vi "Splash Screen.vi"() -> ()   [LabVIEW 2026, in "CI Tests Launcher.lvlib"]
doc: "This is the top-level VI of this application. When it runs, it behaves like the splash screen many applications use to keep the user occupied while the application loads into memory. This application is quite small, so there is little overhead, which would make the splash screen just flash for a moment. Because that flash is distracting, there is a three-second delay inserted into this VI so that it stays up for a little bit. \n\nThis VI uses a delay-loaded subVI call to load the rest of the application. This trick ensures that the splash screen can load instantly regardless of how large the rest of the VI hierarchy gets, and the loading of the rest of the VIs becomes one step in the load process."
uses:
  CI Tests Launcher.lvlib
  CI Tests/CI Tests/Load App.vi
  CI Tests/CI Tests/CI Tests.lvclass
panel:
  out "Waiting Lights":T1
  out "Application Name":string
  out "Current Action":string caption="Current action:"
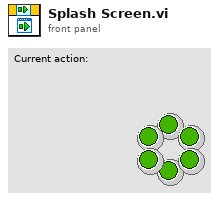
[diagram p1: front panel]
types:
  T1 = cluster{"wait 1":bool, "wait 2":bool, "wait 3":bool, "wait 4":bool, "wait 5":bool, "wait 6":bool}
  T2 = cluster{"[0]":bool, "[1]":bool, "[2]":bool, "[3]":bool, "[4]":bool, "[5]":bool}
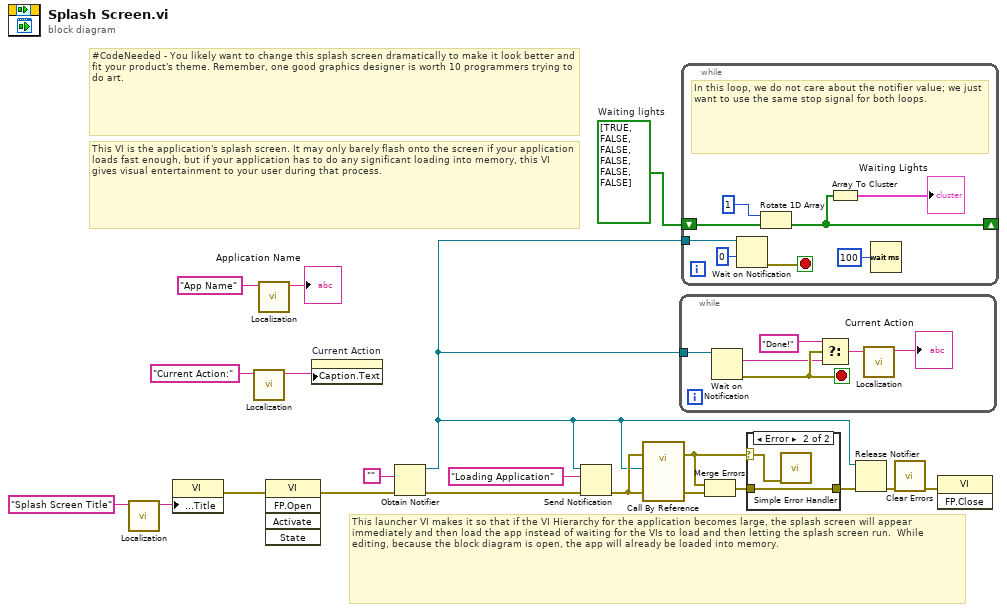
[diagram p0: block diagram]
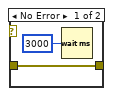
[diagram p2: hidden frame]
diagram:
  w10 = bool[] [TRUE, FALSE, FALSE, FALSE, FALSE, FALSE]  # Waiting lights
  # "#CodeNeeded - You likely want to change this splash screen dramatically to make it look better and fit your product's theme. Remember, one good graphics designer is worth 10 programmers trying to do art."
  # "This VI is the application's splash screen. It may only barely flash onto the screen if your application loads fast enough, but if your application has to do any significant loading into memory, this VI gives visual entertainment to your user during that process."
  # "This launcher VI makes it so that if the VI Hierarchy for the application becomes large, the splash screen will appear immediately and then load the app instead of waiting for the VIs to load and then letting the splash screen run.  While editing, because the block diagram is open, the app will already be loaded into memory."
  n1 = call "Localization.vi"("Unlocalized"="Splash Screen Title" ("Window Title")) -> ("Localized"=w20:string)  [unwired: 10 in]
  n2 = property class="VI"("Front Panel.Title"=w20) -> (error out=w2:errorcluster)  [unwired: 2 in, 1 out]
  n3 = call "Localization.vi"("Unlocalized"="Current Action:" ("Window Title")) -> ("Localized"=w6:string)  [unwired: 10 in]
  n4 = call "Localization.vi"("Unlocalized"="App Name") -> ("Localized"=→"Application Name":string)  [unwired: 10 in]
  n5 = invoke class="VI" method="FP.Open"(error in=w2) -> (error out=w1:errorcluster)  [unwired: 4 in, 4 out]
  n6 = property on="Current Action" class="Str"("Caption.Text"=w6) -> ()  [unwired: 2 in, 2 out]
  n7 = Obtain Notifier(notification data type="", error in (no error)=w1) -> (notifier out=w14:refnum<notifier>, error out=w8:errorcluster)  [unwired: 2 in, 1 out]
  n8 = Send Notification(notification="Loading Application", notifier=w14, error in (no error)=w8) -> (error out=w15:errorcluster)  [unwired: 1 out]
  n9 = call-by-ref "?"(error in=w15, 8:"error in (no error)"=w15, "Status Notifier"=w14) -> (error out=w3:errorcluster, 0:"error out"=w18:errorcluster)  [unwired: 10 in, 1 out]
  n10 = while {
    tunnel: w14 -> [w25]
    stop <- w24 stop-if-true
    n11 = Wait on Notification(notifier=w25) -> (notification=w22:string, error out=w24:errorcluster)  [unwired: 3 in, 2 out]
    n12 = Select(t="Done!" ("notification"), s=w24, f=w22) -> (s? t:f=w21:string)
    n13 = call "Localization.vi"("Unlocalized"=w21) -> ("Localized"=→"Current Action":string)  [unwired: 10 in]
  }
  n14 = while {
    shift-right: [w28] -> _
    shift-left: w10 -> [w30]
    tunnel: w14 -> [w32]
    stop <- w34 stop-if-true
    # "In this loop, we do not care about the notifier value; we just want to use the same stop signal for both loops."
    n15 = Wait on Notification(notifier=w32, timeout in ms (-1)=0) -> (error out=w34:errorcluster)  [unwired: 2 in, 3 out]
    n16 = Rotate 1D Array(1:w30, 2:1 ("n")) -> (0:w28:bool[])
    n17 = Array To Cluster(array=w28) -> (cluster=→"Waiting Lights":T2)
    n18 = Wait (ms)(milliseconds to wait=u32 100) -> ()  [unwired: 1 out]
  }
  n19 = Merge Errors(w3, w18) -> (w4:errorcluster)
  n20 = case shown="Error" w3 {
    tunnel: [w36 w37] -> w5
    tunnel: w4 -> [w36 w37]
    selector: w3 -> [_ w38]
    frame No Error {
      n21 = Wait (ms)(milliseconds to wait=u32 3000) -> ()  [unwired: 1 out]
    }
    frame Error {
      n22 = call <vilib>:"Simple Error Handler.vi"("error in (no error)"=w38) -> ()  [unwired: 4 in, 5 out]
    }
  }
  n23 = Release Notifier(notifier=w14, error in (no error)=w5) -> (error out=w17:errorcluster)  [unwired: 1 in, 2 out]
  n24 = call <vilib>:"Clear Errors.vi"("error in (no error)"=w17) -> ("error out"=w9:errorcluster)  [unwired: 5 in, 1 out]
  n25 = invoke class="VI" method="FP.Close"(error in=w9) -> ()  [unwired: 2 in, 3 out]
